vi "valve_queue.vi"() -> (0 "error out":errorcluster, 3 "Queue out":refnum<queue>)   [LabVIEW 2013]
uses:
  type_defs/valve_message.ctl
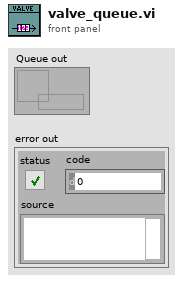
[diagram p1: front panel]
types:
  T1 = typedef "valve_message.ctl" = enum16{"INITALIZE", "MOVE TO NEXT VALVE"}
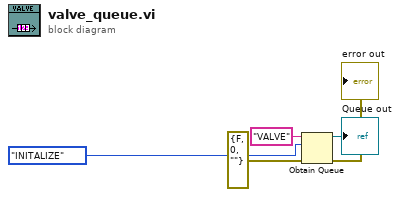
[diagram p0: block diagram]
diagram:
  n1 = Obtain Queue(name (unnamed)="VALVE", element data type=valve_message."INITALIZE", error in (no error)=errorcluster {"status"=FALSE, "code"=0, "source"=""}) -> (queue out=→"Queue out":refnum<queue>, error out=→"error out":errorcluster)  [unwired: 2 in, 1 out]
